vi "Async File Reader.vi"() -> ()   [LabVIEW 2011, in "Interpolate 1D Array Custom Device.lvlib"]
doc: "This VI which waits on the 'Command FIFO' and then re-reads the spreadsheet and brings the new data back via the 'New Values FIFO'."
uses:
  Interpolate 1D Array Custom Device.lvlib
  <vilib>/NI Veristand/Custom Device API/Custom Device Item Ref.ctl
  <vilib>/NI Veristand/Custom Device API/Custom Device API.lvlib
panel:
  out "Y Array":dbl[](array[numeric])
  out "X Array":dbl[](array[numeric])
  out "element out":bool
  in  "Input Data":T2 {"Device Reference in" format="%.0x"}
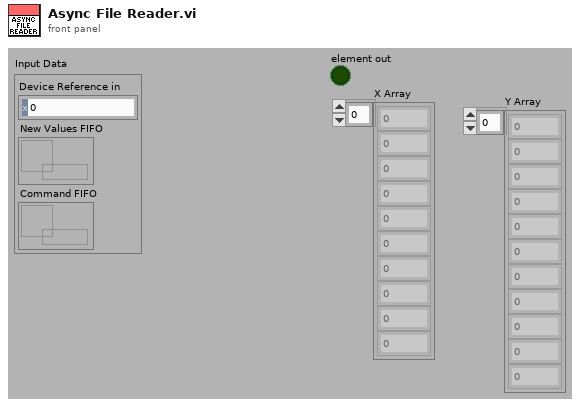
[diagram p1: front panel]
types:
  T1 = typedef "Custom Device API.lvlib/Custom Device Item Ref.ctl" = u64
  T2 = cluster{"Device Reference in":T1, "New Values FIFO":refnum<k33>, "Command FIFO":refnum<k33>}
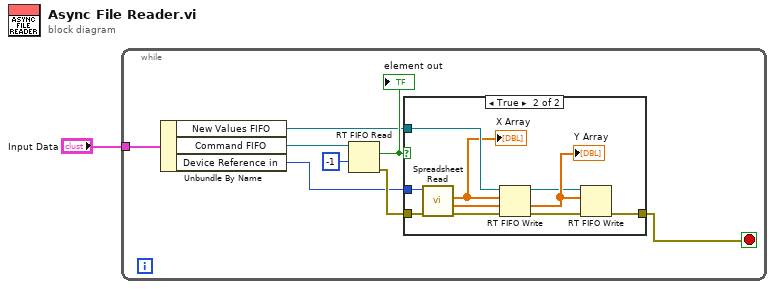
[diagram p0: block diagram]
diagram:
  n1 = while {
    tunnel: "Input Data" -> [w8]
    stop <- w6 stop-if-true
    n2 = Unbundle By Name(w8) -> ("New Values FIFO"=w4:refnum<k33>, "Command FIFO"=w3:refnum<k33>, "Device Reference in"=w2:T1)
    n3 = RT FIFO Read(0:w3, 2:-1 ("timeout in ms (0)")) -> (9:w9:bool, 11:w7:errorcluster)  [unwired: 2 in, 3 out]
    "element out" <- w9
    n4 = case shown="True" w9 {
      tunnel: w4 -> [_ w17]
      tunnel: w2 -> [_ w14]
      tunnel: w7 -> [w10 w13]
      tunnel: [w10 w12] -> w6
      frame False {
      }
      frame True {
        n5 = call "Spreadsheet Read.vi"("error in (no error)"=w13, "Device Reference in"=w14) -> ("error out"=w15:errorcluster, "Y Array"=w19:dbl[], "X Array"=w11:dbl[])  [unwired: 6 in, 1 out]
        "Y Array" <- w19
        "X Array" <- w11
        n6 = RT FIFO Write(0:w17, 1:w11, 3:w15) -> (8:w18:refnum<k33>, 11:w16:errorcluster)  [unwired: 2 in, 2 out]
        n7 = RT FIFO Write(0:w18, 1:w19, 3:w16) -> (11:w12:errorcluster)  [unwired: 2 in, 3 out]
      }
    }
  }
